vi "NI Timing Card.vi"() -> ()   [LabVIEW 2015]
uses:
  SubVIs/State Control.ctl
panel:
  in  "Repeat":bool
  out "Master Timebase":dbl[unit]=100000000.0 format="%#_6p"
  in  "Start":bool
  in  "Counters":T1(array[cluster])=[{"Counter"=1, "Delay"=1.0, "Mode"=enum."Rising Edge", "Pulse Width"=0.0}, {"Counter"=2, "Delay"=1.0, "Mode"=enum."Rising Edge", "Pulse Width"=0.0}, {"Counter"=3, "Delay"=1.0, "Mode"=enum."Rising Edge", "Pulse Width"=0.0}, {"Counter"=4, "Delay"=1.0, "Mode"=enum."Rising Edge", "Pulse Width"=0.0}] {"Pulse Width" format="%.6p"; "Delay" format="%.6p"; "Counter" items=["ctr0", "ctr1", "ctr2", "ctr3", "ctr4", "ctr5", "ctr6", "ctr7"]}
  in  "Measurment Time":dbl[unit]=5.0 format="%.6p"
  in  "Pre-Trigger Time":dbl[unit]=1.0 format="%.6p"
  in  "Master Counter":tag="6612/ctr0"
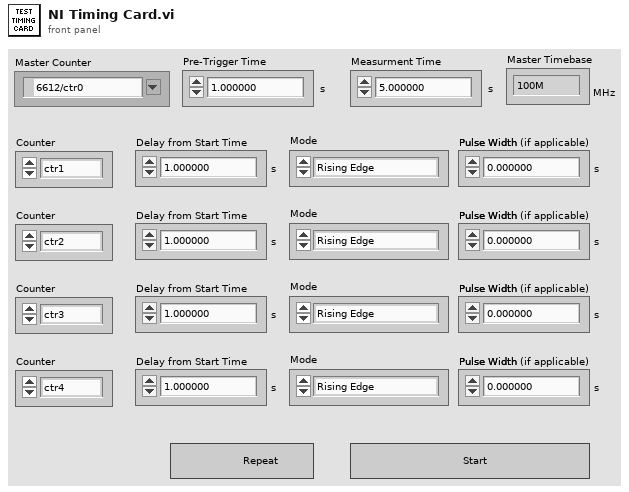
[diagram p1: front panel]
types:
  T1 = cluster{"Counter":u16, "Delay":dbl[unit], "Mode":enum16{"Rising Edge", "Falling Edge", "High Going Pulse", "Low Going Pulse"}, "Pulse Width":dbl[unit]}[]
  T2 = typedef "State Control.ctl" = enum16{"Setup Tasks", "Handle UI Events", "Run Tasks"}
  T3 = enum8{"Enabled", "Disabled", "Disabled and Grayed Out"}
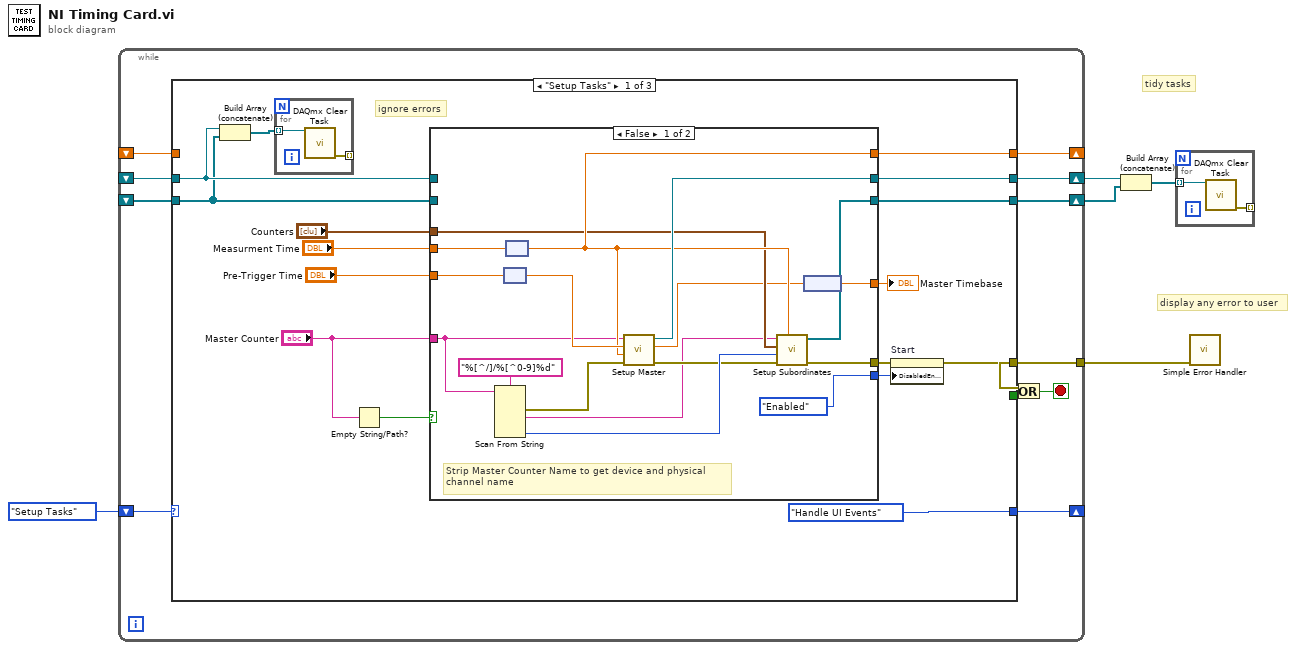
[diagram p0: block diagram]
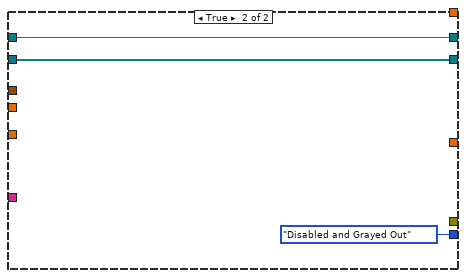
[diagram p2: hidden frame]
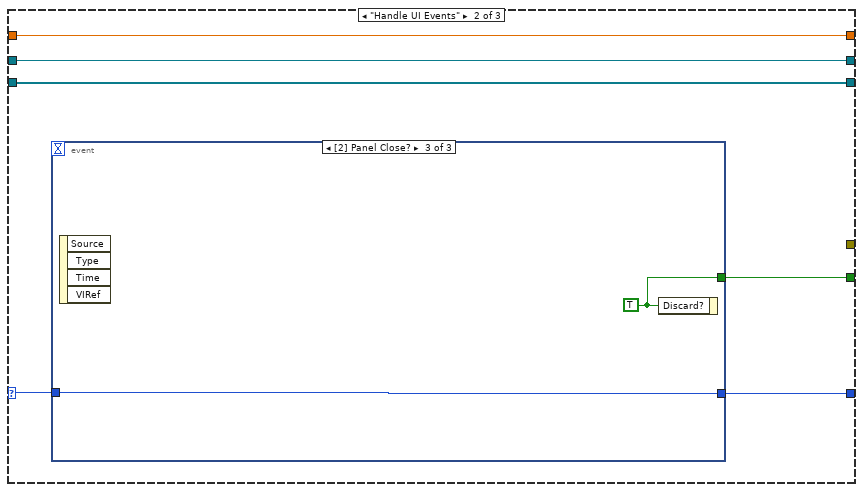
[diagram p3: hidden frame]
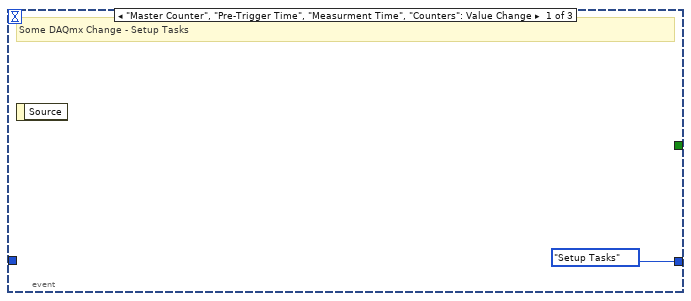
[diagram p4: hidden frame]
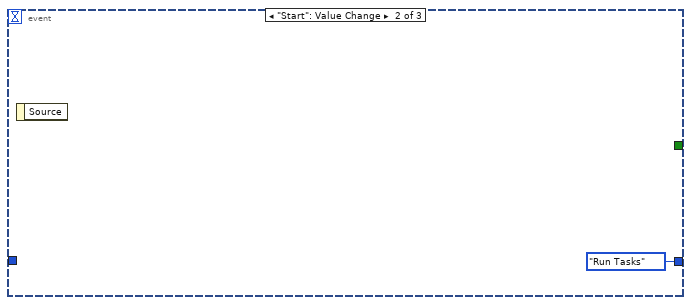
[diagram p5: hidden frame]
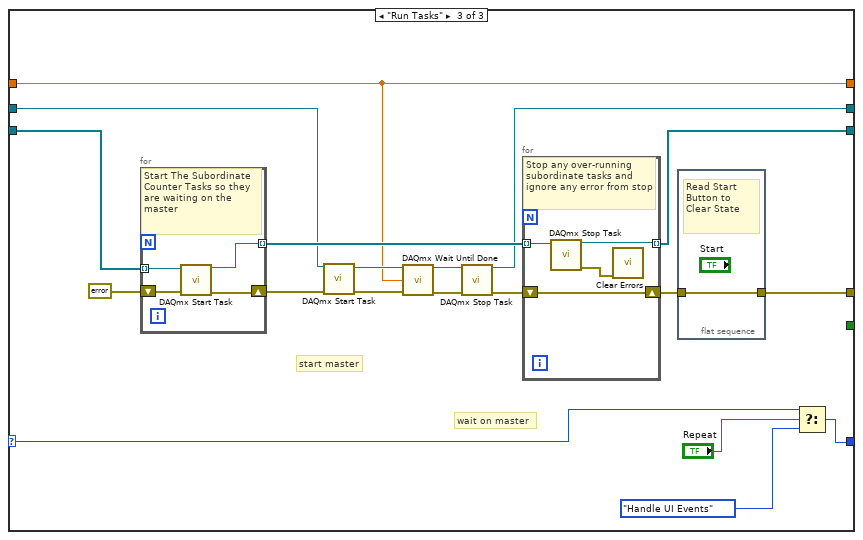
[diagram p6: hidden frame]
diagram:
  # "tidy tasks"
  # "display any error to user"
  n1 = while {
    tunnel: [w8] -> w1
    shift-right: [w9] -> _
    shift-left: State_Control."Setup Tasks" ("State") -> [w13]
    shift-right: [w15] -> w3
    shift-left: _ -> [w12]
    shift-right: [w16] -> w2
    shift-left: _ -> [w11]
    shift-right: [w14] -> _
    shift-left: _ -> [w10]
    stop <- w7 stop-if-true
    n2 = case shown="\"Setup Tasks\"" w13 {
      selector: w13 -> [_ w55 w67]
      tunnel: [w22 _ w76] -> w8
      tunnel: [w30 w59 w69] -> w16
      tunnel: [w29 w60 w73] -> w15
      tunnel: [w28 w58 w78] -> w14
      tunnel: w12 -> [w21 w60 w79]
      tunnel: w11 -> [w20 w59 w70]
      tunnel: w10 -> [_ w58 w78]
      tunnel: [State_Control."Handle UI Events" ("State") w57 w66] -> w9
      tunnel: [_ w56 _] -> w6
      frame "Setup Tasks" {
        # "ignore errors"
        n3 = Build Array (concatenate)(w21, w20) -> (w19:refnum<k21>[])
        n4 = for {
          tunnel: w19 -> [w34] mode=indexing
          tunnel: [w33] -> _ mode=indexing
          n5 = call <vilib>:"DAQmx Clear Task.vi"("task in"=w34) -> ("error out"=w33:errorcluster)  [unwired: 14 in]
        }
        n6 = Empty String/Path?(string/path="Master Counter") -> (empty?=w24:bool)
        n7 = case shown="False" w24 {
          tunnel: "Pre-Trigger Time" -> [w51 _]
          tunnel: "Measurment Time" -> [w50 _]
          tunnel: [w46 _] -> w23
          tunnel: [w45 w53] -> w30
          tunnel: [w44 w54] -> w29
          tunnel: [w41 _] -> w28
          tunnel: "Counters" -> [w40 _]
          tunnel: "Master Counter" -> [w38 _]
          tunnel: w21 -> [_ w54]
          tunnel: w20 -> [_ w53]
          tunnel: [T3."Enabled" ("Disabled") T3."Disabled and Grayed Out" ("Disabled")] -> w18
          tunnel: [w35 _] -> w17
          frame False {
            # "Strip Master Counter Name to get device and physical\nchannel name"
            n8 = Scan From String(format string="%[^/]/%[^0-9]%d", input string=w38) -> (error out=w48:errorcluster, output 1=w39:string, output 3=w47:i32)  [unwired: 6 in, 2 out]
            n9 = node(w51) -> (w42:dbl)
            n10 = node(w50) -> (w41:dbl)
            n11 = call "Setup Master.vi"("error in (no error)"=w48, "Measurment Time(s)"=w41, "Pre-Trigger Time(s)"=w42, "Master Counter"=w38) -> ("error out"=w43:errorcluster, "Master Timebase"=w36:dbl, "Master Task out"=w44:refnum<k21>)  [unwired: 5 in]
            n12 = call "Setup Subordinates.vi"("Measurment Duration (s)"=w41, "error in (no error)"=w43, "Master Counter#"=w47, "Counters"=w40, "Device Name"=w39) -> ("error out"=w46:errorcluster, "Array"=w45:refnum<k21>[])  [unwired: 5 in]
            n13 = node(w36) -> (w35:dbl[unit])
          }
          frame True {
          }
        }
        "Master Timebase" <- w17
        n14 = property on="Start" class="Bool"(error in=w23, "DisabledEnum"=w18) -> (error out=w22:errorcluster)  [unwired: 1 in, 1 out]
      }
      frame "Handle UI Events" {
        n15 = event shown="[2] Panel Close?" {
          selector: _ -> [_ _ _]
          dyn-events: _ -> [_ _ _]
          timeout: _ -> [_ _ _]
          tunnel: [State_Control."Setup Tasks" ("State") State_Control."Run Tasks" ("State") w63] -> w57
          tunnel: [_ _ w64] -> w56
          tunnel: w55 -> [_ _ w63]
          event "Master Counter", "Pre-Trigger Time", "Measurment Time", "Counters": Value Change {
            # "Some DAQmx Change - Setup Tasks"
            n16 = event-data() -> ()  [unwired: 1 in, 1 out]
          }
          event "Start": Value Change {
            n17 = event-data() -> ()  [unwired: 1 in, 1 out]
          }
          event Panel Close? {
            w64 = TRUE ("Discard?")
            n18 = event-data() -> ()  [unwired: 1 in, 4 out]
            n19 = event-data("Discard?"=w64) -> ()  [unwired: 1 in, 1 out]
          }
        }
      }
      frame "Run Tasks" {
        # "wait on master"
        # "start master"
        n20 = for {
          tunnel: w70 -> [w92] mode=indexing
          shift-right: [w90] -> w80
          shift-left: errorcluster {"status"=FALSE, "code"=0, "source"=""} ("error out") -> [w91]
          tunnel: [w89] -> w83 mode=indexing
          # "Start The Subordinate Counter Tasks so they are waiting on the master"
          n21 = call <vilib>:"DAQmx Start Task.vi"("task/channels in"=w92, "error in"=w91) -> ("task out"=w89:refnum<k21>, "error out"=w90:errorcluster)  [unwired: 12 in]
        }
        n22 = call <vilib>:"DAQmx Start Task.vi"("task/channels in"=w79, "error in"=w80) -> ("task out"=w82:refnum<k21>, "error out"=w81:errorcluster)  [unwired: 12 in]
        n23 = call <vilib>:"DAQmx Wait Until Done.vi"("task/channels in"=w82, "timeout (sec)"=w78, "error in"=w81) -> ("task out"=w77:refnum<k21>, "error out"=w72:errorcluster)  [unwired: 11 in]
        n24 = call <vilib>:"DAQmx Stop Task.vi"("task/channels in"=w77, "error in"=w72) -> ("task out"=w73:refnum<k21>, "error out"=w71:errorcluster)  [unwired: 12 in]
        n25 = for {
          tunnel: w83 -> [w88] mode=indexing
          shift-right: [w87] -> w75
          shift-left: w71 -> [w87]
          tunnel: [w86] -> w69 mode=indexing
          # "Stop any over-running subordinate tasks and ignore any error from stop"
          n26 = call <vilib>:"DAQmx Stop Task.vi"("task/channels in"=w88) -> ("task out"=w86:refnum<k21>, "error out"=w85:errorcluster)  [unwired: 13 in]
          n27 = call <vilib>:"Clear Errors.vi"("error in (no error)"=w85) -> ()  [unwired: 5 in, 2 out]
        }
        n28 = flat-sequence {
          tunnel: [w84] -> w76
          tunnel: w75 -> [w84]
          frame #0 {
            # "Read Start Button to Clear State"
          }
        }
        n29 = Select(t=w67, s="Repeat", f=State_Control."Handle UI Events" ("State")) -> (s? t:f=w66:T2)
      }
    }
    n30 = Or(x=w8, y=w6) -> (x .or. y?=w7:bool)
  }
  n31 = Build Array (concatenate)(w3, w2) -> (w4:refnum<k21>[])
  n32 = for {
    tunnel: w4 -> [w94] mode=indexing
    tunnel: [w93] -> _ mode=indexing
    n33 = call <vilib>:"DAQmx Clear Task.vi"("task in"=w94) -> ("error out"=w93:errorcluster)  [unwired: 14 in]
  }
  n34 = call <vilib>:"Simple Error Handler.vi"("error in (no error)"=w1) -> ()  [unwired: 4 in, 5 out]
